vi "MP-285 Get Position.vi"(5 "error in (no error)":errorcluster, 6 "VISA resource name":refnum<visa-resource-name>) -> (0 "error out":errorcluster, 1 "Output: Z axis (microns)":dbl format="%.2f", 2 "Output: Y axis (microns)":dbl format="%.2f", 3 "Output: X axis (microns)":dbl format="%.2f", 4 "VISA resource name out":refnum<visa-resource-name>)   [LabVIEW 2010]
panel:
  out "Serial Read":string
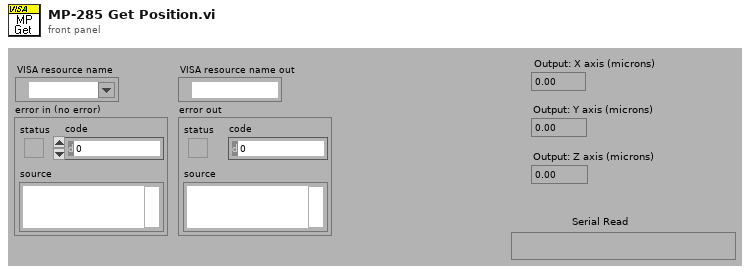
[diagram p1: front panel]
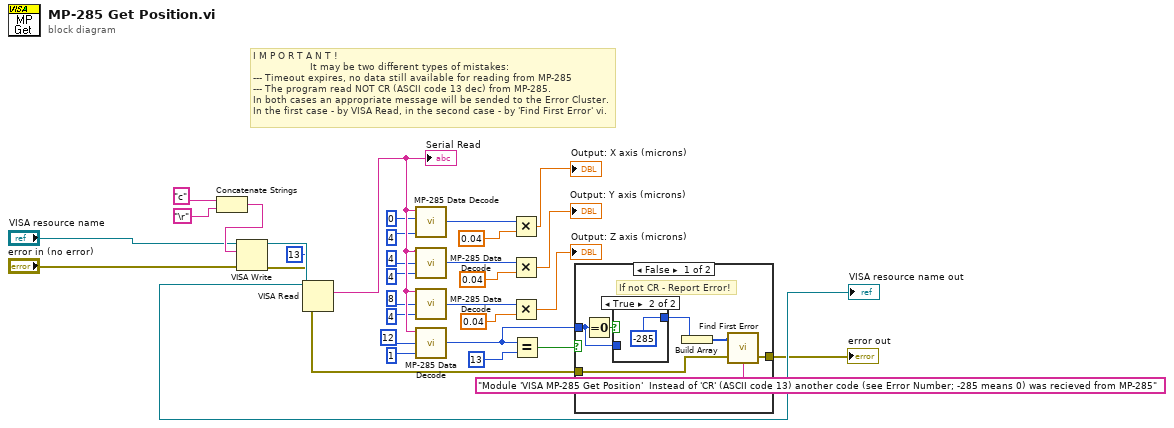
[diagram p0: block diagram]
diagram:
  # "I M P O R T A N T !\n                   It may be two different types of mistakes: \n--- Timeout expires, no data still available for reading from MP-285\n--- The program read NOT CR (ASCII code 13 dec) from MP-285.\nIn both cases an appropriate message will be sended to the Error Cluster.\nIn the first case - by VISA Read, in the second case - by 'Find First Error' vi."
  n1 = Concatenate Strings("c", "\r") -> (w24:string)
  n2 = VISA Write(VISA resource name="VISA resource name", write buffer=w24, error in (no error)="error in (no error)") -> (VISA resource name out=w23:refnum<visa-resource-name>, error out=w22:errorcluster)  [unwired: 1 out]
  n3 = VISA Read(VISA resource name=w23, byte count=13, error in (no error)=w22) -> (VISA resource name out=→"VISA resource name out":refnum<visa-resource-name>, read buffer=w12:string, error out=w14:errorcluster)  [unwired: 1 out]
  "Serial Read" <- w12
  n4 = call "MP-285 Data Decode.vi"("Input: lenght"=4 ("length"), "Input: offset"=0 ("offset (0)"), "Input: Data string"=w12) -> ("Output: Decoded Data"=w32:i32)
  n5 = call "MP-285 Data Decode.vi"("Input: lenght"=4 ("length"), "Input: offset"=4 ("offset (0)"), "Input: Data string"=w12) -> ("Output: Decoded Data"=w28:i32)
  n6 = call "MP-285 Data Decode.vi"("Input: lenght"=4 ("length"), "Input: offset"=8 ("offset (0)"), "Input: Data string"=w12) -> ("Output: Decoded Data"=w29:i32)
  n7 = call "MP-285 Data Decode.vi"("Input: lenght"=1, "Input: offset"=12, "Input: Data string"=w12) -> ("Output: Decoded Data"=w15:i32)
  n8 = Multiply(x=w32, y=0.04) -> (x*y=→"Output: X axis (microns)":dbl)
  n9 = Multiply(x=w28, y=0.04) -> (x*y=→"Output: Y axis (microns)":dbl)
  n10 = Multiply(x=w29, y=0.04) -> (x*y=→"Output: Z axis (microns)":dbl)
  n11 = Equal?(x=w15, y=13) -> (x = y?=w16:bool)
  n12 = case shown="False" w16 {
    tunnel: [w39 w42] -> w1
    tunnel: w15 -> [w34 _]
    tunnel: w14 -> [w36 w42]
    frame False {
      # "If not CR - Report Error!"
      n13 = Equal To 0?(x=w34) -> (x = 0?=w35:bool)
      n14 = case shown="True" w35 {
        tunnel: w34 -> [w40 _]
        tunnel: [w40 -285] -> w33
        frame False {
        }
        frame True {
        }
      }
      n15 = Build Array(w33) -> (w37:i32[])
      n16 = call <vilib>:"Find First Error.vi"("error in (no error)"=w36, "source messages"="Module 'VISA MP-285 Get Position'  Instead of 'CR' (ASCII code 13) another code (see Error Number; -285 means 0) was recieved from MP-285", "error codes"=w37) -> ("error out"=w39:errorcluster)  [unwired: 2 out]
    }
    frame True {
      # "The CR was readed\n        NO Errors"
      # "TRUE CR was received - NO Errors"
    }
  }
  "error out" <- w1
